vi "Test View get View VI Reference.vi"(8 "error in (no error)":errorcluster, 11 "View Test In":refnum<class "View Test.lvclass">) -> (0 "error out":errorcluster, 3 "View Test Out":refnum<class "View Test.lvclass">)   [LabVIEW 2020, in "View Test.lvclass"]
uses:
  View Test.lvclass
  Framework/View/View.lvclass
  <vilib>/Asteme/LUnit/Test Case.lvclass
  C:/Users/anton/Documents/GitHub/Triarc-Framework/source/Framework Test/Process Test/Process Test.lvclass
  C:/Users/anton/Documents/GitHub/Triarc-Framework/source/Framework Test/Base Class Test/Base Test.lvclass
  C:/Program Files (x86)/National Instruments/LabVIEW 2020/vi.lib/Asteme/LUnit/Test Case.lvclass
  C:/Users/anton/Documents/GitHub/Triarc-Framework/source/Framework Test/View Test/View Test.lvclass
  Framework/Process/Process.lvclass
  C:/Users/anton/Documents/GitHub/Triarc-Framework/source/Framework/Process/Process.lvclass
  C:/Users/anton/Documents/GitHub/Triarc-Framework/source/Framework/Base/Base.lvclass
  C:/Users/anton/Documents/GitHub/Triarc-Framework/source/Framework/Configuration File/Configuration File.lvclass
  C:/Users/anton/Documents/GitHub/Triarc-Framework/source/Framework/Error Handler Interface/Error Handler Interface.lvclass
  C:/Users/anton/Documents/GitHub/Triarc-Framework/source/Framework/View/View.lvclass
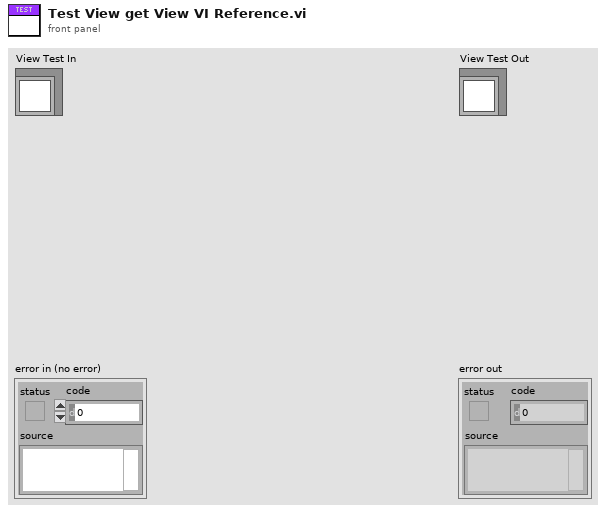
[diagram p1: front panel]
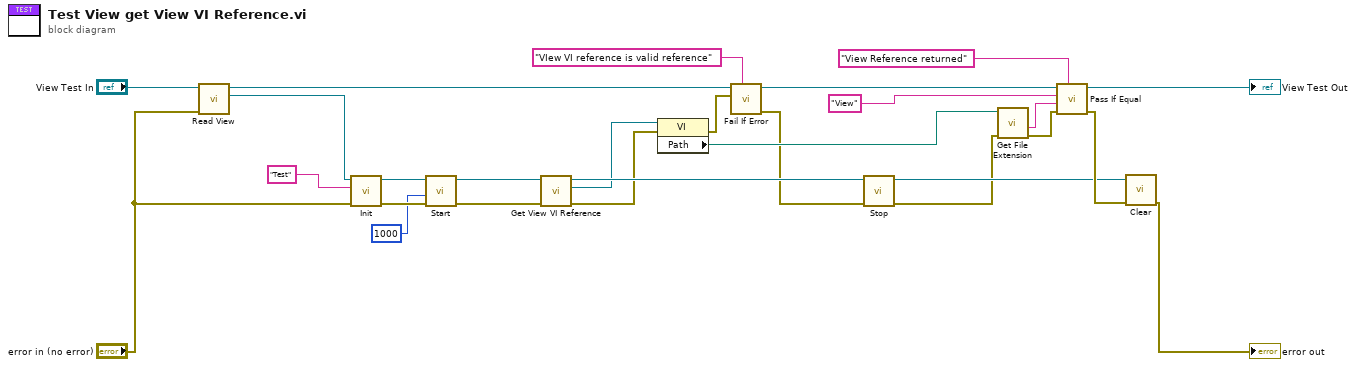
[diagram p0: block diagram]
diagram:
  n1 = call "Read View.vi"("error in (no error)"="error in (no error)", "View Test In"="View Test In") -> ("View"=w26:refnum<class "View.lvclass">, "View Test Out"=w27:refnum<class "View Test.lvclass">)  [unwired: 7 in, 1 out]
  n2 = call-dynamic "Init.vi"("error in (no error)"="error in (no error)", "Name"="Test", "View In"=w26) -> ("error out"=w17:errorcluster, "View Out"=w18:refnum<class "View.lvclass">)  [unwired: 7 in]
  n3 = call "Start.vi"("error in (no error)"=w17, "Timeout [ms] (-1)"=1000, "Process In"=w18) -> ("error out"=w12:errorcluster, "Process Out"=w13:refnum<class "View.lvclass">)  [unwired: 7 in]
  n4 = call "Get View VI Reference.vi"("error in (no error)"=w12, "UI View In"=w13) -> ("error out"=w5:errorcluster, "View VI Reference"=w11:refnum<vi>, "UI View Out"=w16:refnum<class "View.lvclass">)  [unwired: 7 in]
  n5 = property class="VI"(reference=w11, error in=w5) -> (error out=w4:errorcluster, "Path"=w10:path)  [unwired: 1 out]
  n6 = call <vilib>:"Fail If Error.vi"("Description"="VIew VI reference is valid reference", "Assert error"=w4, "Test Case In"=w27) -> ("error out"=w2:errorcluster, "Test Case Out"=w6:refnum<class "View Test.lvclass">)  [unwired: 7 in]
  n7 = call "Stop.vi"("error in (no error)"=w2, "Process In"=w16) -> ("error out"=w14:errorcluster, "Process Out"=w15:refnum<class "View.lvclass">)  [unwired: 7 in, 1 out]
  n8 = call <vilib>:"Get File Extension.vi"("error in (no error)"=w14, "file"=w10) -> ("error out"=w7:errorcluster, "filename without extension"=w9:string)  [unwired: 5 in, 3 out]
  n9 = call <vilib>:"Pass If Equal.vi"("Description"="View Reference returned", "error in (no error)"=w7, "Actual"=w9, "Expected"="View", "Test Case In"=w6) -> ("error out"=w25:errorcluster, "Test Case Out"=→"View Test Out":refnum<class "View Test.lvclass">)  [unwired: 5 in]
  n10 = call-dynamic "Clear.vi"("error in (no error)"=w25, "View In"=w15) -> ("error out"=→"error out":errorcluster)  [unwired: 8 in, 1 out]
